vi "test Cluster UserEvent.vi"() -> ()   [LabVIEW 2023]
uses:
  target/debug/liblabview_test_library.dylib
panel:
  out "error out":errorcluster
  out "return type":i32
  out "id":string
  out "eventno":i32
  in  "Running":bool=TRUE
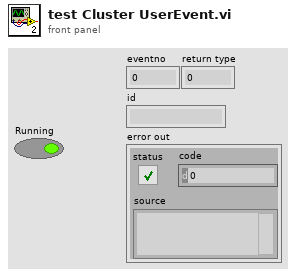
[diagram p1: front panel]
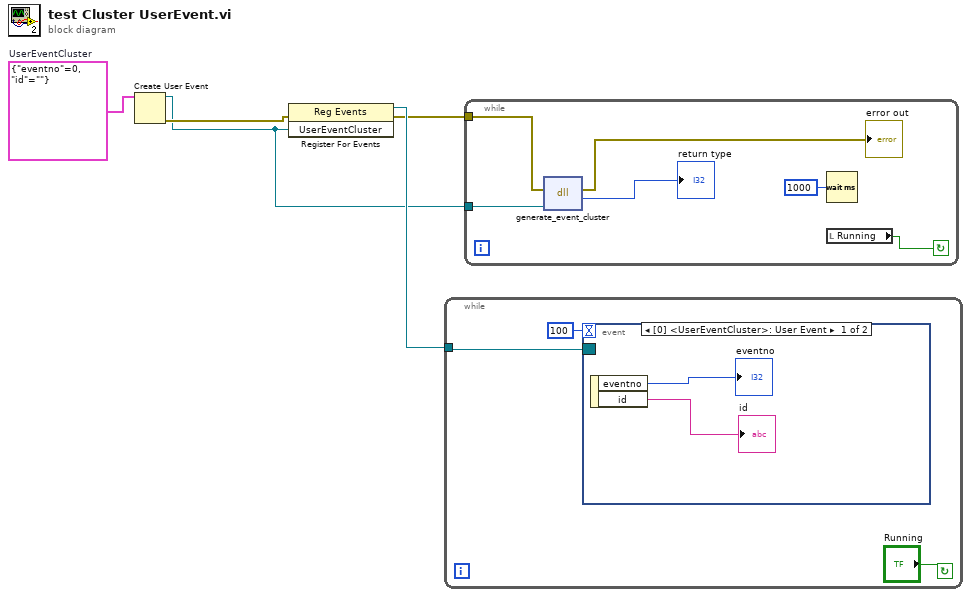
[diagram p0: block diagram]
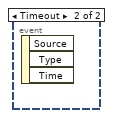
[diagram p2: hidden frame]
diagram:
  w5 = cluster{"eventno":i32, "id":string} {"eventno"=0, "id"=""}  # UserEventCluster
  n1 = Create User Event(user event datatype=w5) -> (user event=w1:refnum<user-event>, error out=w4:errorcluster)  [unwired: 1 in]
  n2 = register-events(error in=w4, w1) -> (reference out=w3:refnum<event-registration>, error out=w2:errorcluster)  [unwired: 1 in]
  n3 = while {
    tunnel: w3 -> [w7]
    stop <- "Running" continue-if-true
    n4 = event shown="[0] <UserEventCluster>: User Event" {
      selector: w7 -> [_ _]
      dyn-events: _ -> [_ _]
      timeout: 100 -> [_ _]
      event User Event {
        n5 = event-data() -> ("eventno"=→"eventno":i32, "id"=→"id":string)  [unwired: 1 in]
      }
      event Timeout {
        n6 = event-data() -> ()  [unwired: 1 in, 3 out]
      }
    }
  }
  n7 = while {
    tunnel: w2 -> [w14]
    tunnel: w1 -> [w11]
    stop <- w16 continue-if-true
    n8 = dll-call lib="Volumes/NuFlo/work/src/Rust-LabVIEW-Interop/target/debug/liblabview_test_library.dylib" fn="generate_event_cluster"(error in=w14, "UserEvent"=w11) -> (error out=→"error out":errorcluster, "return type"=→"return type":i32)  [unwired: 3 in, 1 out]
    n9 = Wait (ms)(milliseconds to wait=u32 1000) -> ()  [unwired: 1 out]
    n10 = local read "Running"() -> (w16:bool)
  }
